vi "Configure Power.vi"(8 "error in (no error)":errorcluster, 10 "Power [dBm]":dbl, 11 "VNA-PNA in":refnum<class "VNA-PNA.lvclass">) -> (0 "error out":errorcluster, 3 "VNA-PNA out":refnum<class "VNA-PNA.lvclass">)   [LabVIEW 2020, in "VNA-PNA.lvclass"]
doc: "Configure the output power.\nThe power will be corrected to the nearest supported."
uses:
  VNA-PNA.lvclass
  C:/Sandbox/Git_Sandbox/WiSpry Test Framework source code (LV20)/WiSpry Test Framework/Instruments/Instrument.lvclass
  C:/Sandbox/Git_Sandbox/WiSpry Test Framework source code (LV20)/WiSpry Test Framework/Instruments/Vector Network Analyzer/Vector Network Analyzer.lvclass
  Instrument.lvclass/Instrument.ctl
  Vector Network Analyzer.lvclass/Vector Network Analyzer.ctl
  Instrument.lvclass
  Vector Network Analyzer.lvclass
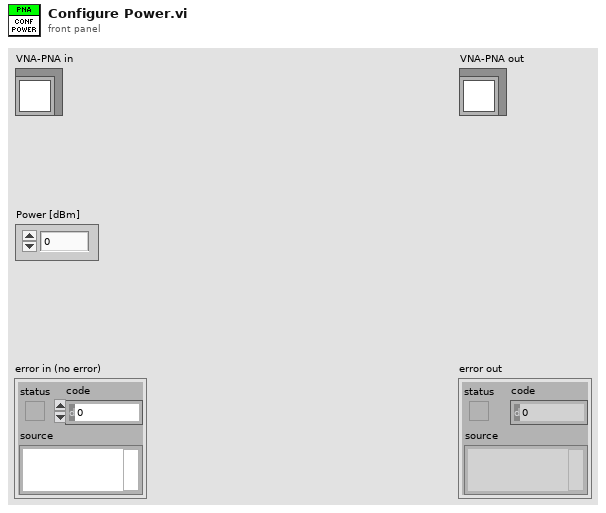
[diagram p1: front panel]
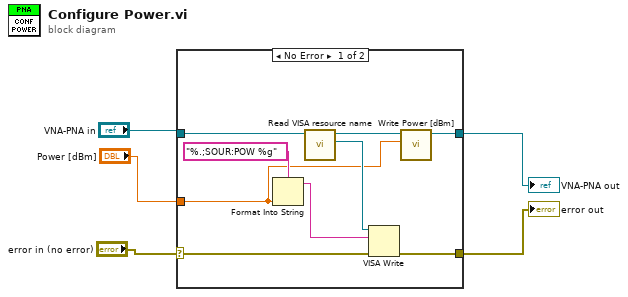
[diagram p0: block diagram]
diagram:
  n1 = case shown="No Error" "error in (no error)" {
    selector: "error in (no error)" -> [w12 w15]
    tunnel: "Power [dBm]" -> [w8 _]
    tunnel: "VNA-PNA in" -> [w13 w16]
    tunnel: [w7 w16] -> w1
    tunnel: [w6 w15] -> w2
    frame No Error {
      n2 = Format Into String(format string="%.;SOUR:POW %g", w8) -> (resulting string=w10:string)  [unwired: 2 in, 1 out]
      n3 = call "Read VISA resource name.vi"("Instrument in"=w13) -> ("VISA resource name"=w11:refnum<visa-resource-name>, "Instrument out"=w9:refnum<class "VNA-PNA.lvclass">)  [unwired: 9 in]
      n4 = VISA Write(VISA resource name=w11, write buffer=w10, error in (no error)=w12) -> (error out=w6:errorcluster)  [unwired: 2 out]
      n5 = call "Write Power [dBm].vi"("Power [dBm]"=w8, "Vector Network Analyzer in"=w9) -> ("Vector Network Analyzer out"=w7:refnum<class "VNA-PNA.lvclass">)  [unwired: 9 in]
    }
    frame Error {
    }
  }
  "error out" <- w2
  "VNA-PNA out" <- w1
